vi "unmarshalling.vi"(7 "Type":variant, 8 "error in (no error)":errorcluster, 10 "String":string, 11 "CustomFlat in":refnum<class "CustomFlat.lvclass">) -> (0 "error out":errorcluster, 2 "Variant":variant, 3 "CustomFlat out":refnum<class "CustomFlat.lvclass">)   [LabVIEW 2023, in "CustomFlat.lvclass"]
uses:
  CustomFlat.lvclass
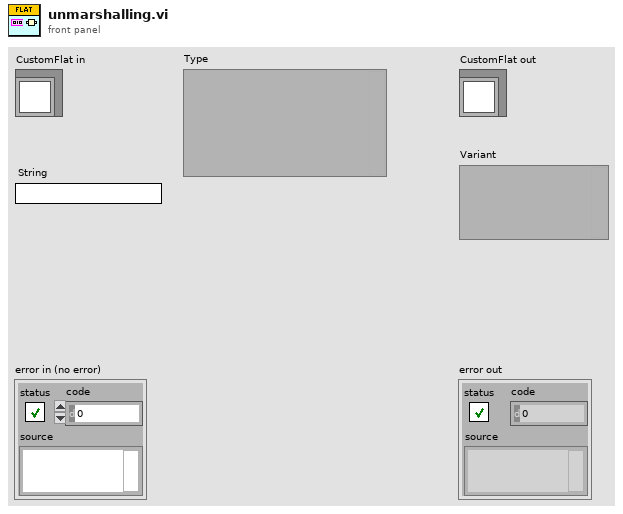
[diagram p1: front panel]
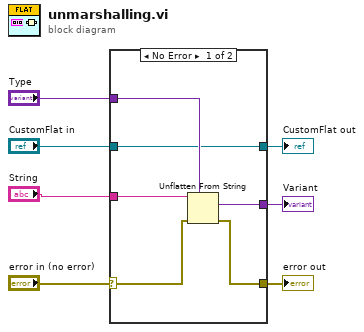
[diagram p0: block diagram]
diagram:
  n1 = case shown="No Error" "error in (no error)" {
    selector: "error in (no error)" -> [w9 w15]
    tunnel: "String" -> [w13 _]
    tunnel: "Type" -> [w12 w14]
    tunnel: [w11 w16] -> w4
    tunnel: "CustomFlat in" -> [w11 w16]
    tunnel: [w10 w14] -> w2
    tunnel: [w8 w15] -> w1
    frame No Error {
      n2 = Unflatten From String(type=w12, binary string=w13, error in (no error)=w9) -> (value=w10:variant, error out=w8:errorcluster)  [unwired: 2 in, 1 out]
    }
    frame Error {
    }
  }
  "error out" <- w1
  "CustomFlat out" <- w4
  "Variant" <- w2
